vi "processData.vi"(8 "error in (no error)":errorcluster, 10 "model":refnum<class "Model.lvclass">, 11 "ControlledMotionState in":refnum<class "CompensatorActiveState.lvclass">) -> (0 "error out":errorcluster, 2 "model 2":refnum<class "Model.lvclass">, 3 "ControlledMotionState out":refnum<class "CompensatorActiveState.lvclass">)   [LabVIEW 2013, in "CompensatorActiveState.lvclass"]
uses:
  CompensatorActiveState.lvclass
  Model/Model/Model.lvclass
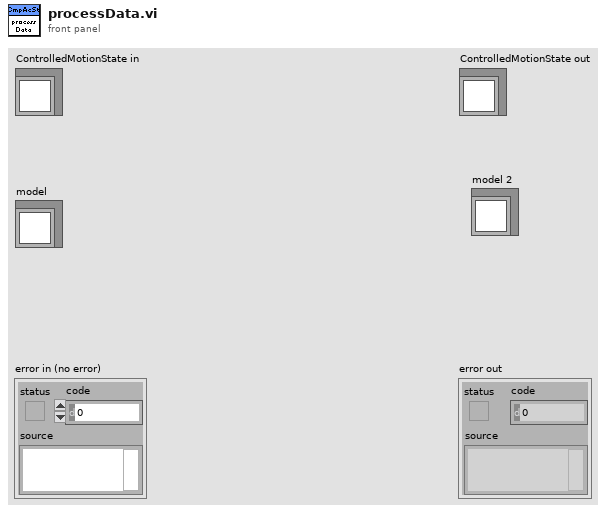
[diagram p1: front panel]
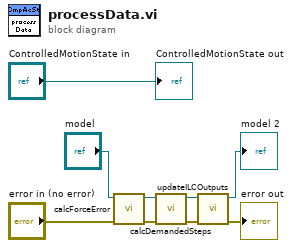
[diagram p0: block diagram]
diagram:
  n1 = call "calcForceError.vi"("error in (no error)"="error in (no error)", "Model in"="model") -> ("error out"=w6:errorcluster, "Model out"=w8:refnum<class "Model.lvclass">)  [unwired: 8 in]
  n2 = call "calcDemandedSteps.vi"("error in (no error)"=w6, "Model in"=w8) -> ("error out"=w4:errorcluster, "Model out"=w5:refnum<class "Model.lvclass">)  [unwired: 8 in]
  n3 = call "updateILCOutputs.vi"("error in (no error)"=w4, "Model in"=w5) -> ("error out"=→"error out":errorcluster, "Model out"=→"model 2":refnum<class "Model.lvclass">)  [unwired: 8 in]
  "ControlledMotionState out" <- "ControlledMotionState in"
